vi "ParseArguments.vi"(8 "error in (no error)":errorcluster, 10 "Inputs":string[](array[string]), 11 "VIPMInstallPackageFile in":refnum<class "VIPMInstallPackageFile.lvclass">) -> (0 "error out":errorcluster, 3 "VIPMInstallPackageFile out":refnum<class "VIPMInstallPackageFile.lvclass">)   [LabVIEW 2014, in "VIPMInstallPackageFile.lvclass"]
uses:
  <nishared>/LabVIEW CLI/Operations/VIPMInstallPackageFile/VIPMInstallPackageFile.lvclass
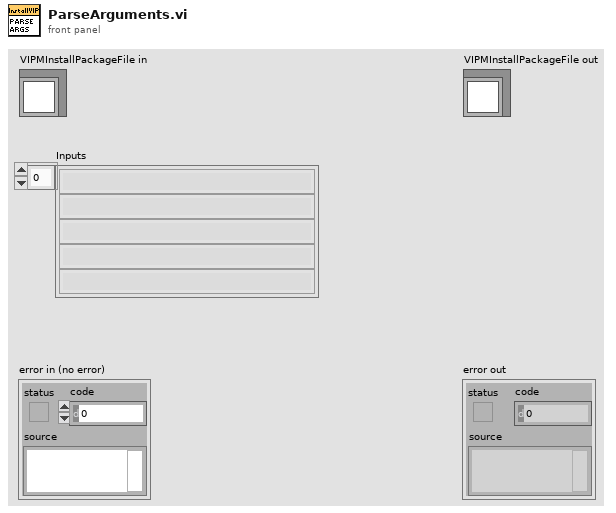
[diagram p1: front panel]
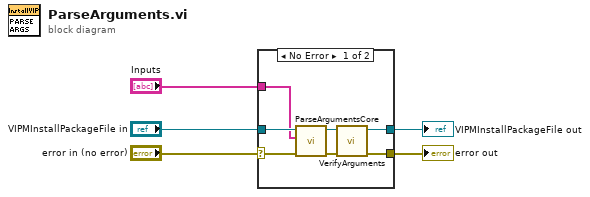
[diagram p0: block diagram]
diagram:
  n1 = case shown="No Error" "error in (no error)" {
    selector: "error in (no error)" -> [w10 w14]
    tunnel: [w8 w14] -> w4
    tunnel: [w6 w13] -> w3
    tunnel: "VIPMInstallPackageFile in" -> [w12 w13]
    tunnel: "Inputs" -> [w11 _]
    frame No Error {
      n2 = call <nishared>:"ParseArgumentsCore.vi"("error in (no error)"=w10, "Inputs"=w11, "VIPMInstallPackageFile in"=w12) -> ("error out"=w9:errorcluster, "VIPMInstallPackageFile out"=w7:refnum<class "VIPMInstallPackageFile.lvclass">)  [unwired: 7 in]
      n3 = call <nishared>:"VerifyArguments.vi"("error in (no error)"=w9, "VIPMInstallPackageFile in"=w7) -> ("error out"=w8:errorcluster, "VIPMInstallPackageFile out"=w6:refnum<class "VIPMInstallPackageFile.lvclass">)  [unwired: 8 in]
    }
    frame Error {
    }
  }
  "error out" <- w4
  "VIPMInstallPackageFile out" <- w3
